vi "Duty Cycle Absolute Encoder.vi"() -> ()   [LabVIEW 2020]
doc: "This example shows how to configure and read values from an absolute encoder that has PWM duty cycle output.\n\nIt will display the raw encoder value, absolute angle, cumulative angle, and revolutions.\n\nThis example expects a USB cable connected from your development PC to the Type B USB Jack (next to the power input) on the roboRIO."
uses:
  <vilib>/Rock Robotics/SystemInterfaces/DIO/FPGA_DIOChannel.ctl
  T-Shirt Robot LV 2020/Shared Code/TypeDefs/ENUM_Tube Wheel Positions.ctl
  T-Shirt Robot LV 2020/roboRIO Code/Type Defs/Cluster_Tube Wheel Positions.ctl
  T-Shirt Robot LV 2020/roboRIO Code/Systems/Tube Wheel/Tube Wheel_ACT.lvlib
panel:
  in  "Position Array":T1[](array[typedef])=[{"Positions"=enum."Tube Red A", "Count"=47}, {"Positions"=enum."Tube Black F", "Count"=213}, {"Positions"=enum."Tube Red E", "Count"=383}, {"Positions"=enum."Tube Black D", "Count"=557}, {"Positions"=enum."Tube Red C", "Count"=724}, {"Positions"=enum."Tube Black B", "Count"=898}]
  out "Current Positions Out":T2
  out "Total Encoder Counts":i32
  out "Total Revolution":dbl
  out "Single Revolution":dbl(knob) scale=0.0..1.0 scale format="%.2g"
  out "Revolutions":i32
  out "Singel Encoder Counts":i32
  in  "Channel":T3=enum."DIO 9"
  in  "stop":bool
  # "Set this input before running."
  # "Output information."
  # "Absolute Encoder\nDuty Cycle (PWM)"
  # "This shows wiring for a generic absolute encoder with duty cycle PWM output.  Some encoders may have G labeled as Com.  Some may have +5V labeled as +VDC."
  # "Encoder\nG (brown wire)--------\n+5V (orange wire)-----\nPWM (blue wire)------"
  # "roboRIO\nDIO-0 \nDIO-0  5V\nDIO-0  S"
  # "PWM"
  # "+5V"
  # "G"
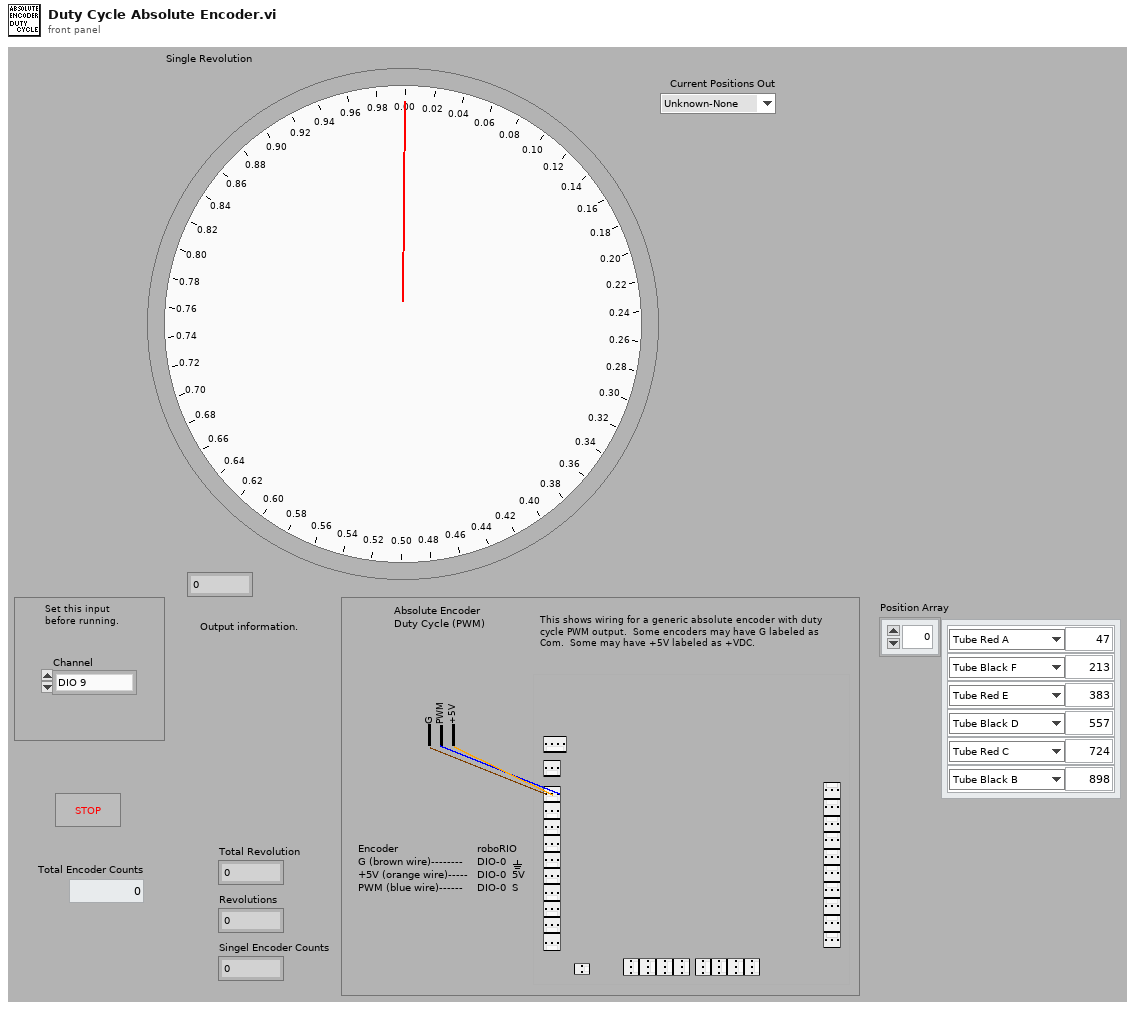
[diagram p1: front panel]
types:
  T1 = typedef "Cluster_Tube Wheel Positions.ctl" = cluster{"Positions":T2, "Count":i32}
  T2 = typedef "ENUM_Tube Wheel Positions.ctl" = enum16{"Unknown-None", "Tube Red A", "Tube Black B", "Tube Red C", "Tube Black D", "Tube Red E", "Tube Black F", "Load A-B", "Load B-C", "Load C-D", "Load D-E", "Load E-F", "Load F-A"}
  T3 = typedef "FPGA_DIOChannel.ctl" = enum8{"DIO 0", "DIO 1", "DIO 2", "DIO 3", "DIO 4", "DIO 5", "DIO 6", "DIO 7", "DIO 8", "DIO 9", "DIO MXP 0", "DIO MXP 1", "DIO MXP 2", "DIO MXP 3", "DIO MXP 4", "DIO MXP 5", "DIO MXP 6", "DIO MXP 7", "DIO MXP 8", "DIO MXP 9", "DIO MXP 10", "DIO MXP 11", "DIO MXP 12", "DIO MXP 13", "DIO MXP 14", "DIO MXP 15", "SPI Port CS1", "SPI Port CS2", "SPI Port CS3", "SPI Port MISO", "SPI Port MOSI", "Invalid"}
  T4 = typedef "Cluster_Absolute Encoder Ref.ctl" = cluster{"DutyCycleDevRef":T5, "CounterDevRef":T7}
  T5 = typedef "FPGA_DutyCycleDevRef.ctl" = cluster{"DevStatus":errorcluster, "DutyCycleIndex":T6}
  T6 = typedef "FPGA_DutyCycleIndex.ctl" = enum8{"DutyCycle 0", "DutyCycle 1", "DutyCycle 2", "DutyCycle 3", "DutyCycle 4", "DutyCycle 5", "DutyCycle 6", "DutyCycle 7", "Invalid"}
  T7 = typedef "WPI_CounterDevRef.ctl" = cluster{"DevStatus":errorcluster, "CntIndex":T8}
  T8 = typedef "FPGA_CounterCtrSystemIndex.ctl" = enum8{"Ctr 0", "Ctr 1", "Ctr 2", "Ctr 3", "Ctr 4", "Ctr 5", "Ctr 6", "Ctr 7", "Invalid"}
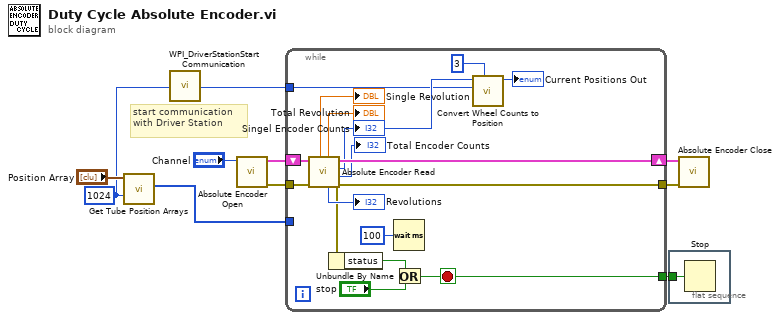
[diagram p0: block diagram]
diagram:
  w1 = 1024 ("PPR")
  # "start communication with Driver Station"
  n1 = call "Get Tube Position Arrays.vi"("PPR"=w1, "Position Array"="Position Array") -> ("Counts"=w2:i32[])  [unwired: 8 in, 1 out]
  n2 = call <vilib>:"WPI_DriverStationStart Communication.vi"() -> ()  [unwired: 3 in, 9 out]
  n3 = call "Absolute Encoder Open.vi"("Channel"="Channel") -> ("error out"=w5:errorcluster, "Cluster"=w7:T4)  [unwired: 9 in]
  n4 = while {
    shift-right: [w18] -> w6
    shift-left: w7 -> [w20]
    tunnel: [w24] -> w8
    tunnel: w5 -> [w19]
    tunnel: [w14] -> w4
    tunnel: w2 -> [_]
    tunnel: w1 -> [w10]
    stop <- w24 stop-if-true
    n5 = call "Absolute Encoder Read.vi"("Error"=w19, "Cluster"=w20) -> ("Error Out"=w14:errorcluster, "Total Encoder Counts Out"=→"Total Encoder Counts":i32, "Single Encoder Counts Out"=w13:i32, "Cluster Out"=w18:T4, "Count Out"=→"Revolutions":i32, "Total Revolution Out"=→"Total Revolution":dbl, "Single Revolution Out"=→"Single Revolution":dbl)  [unwired: 3 in]
    "Singel Encoder Counts" <- w13
    n6 = Unbundle By Name(w14) -> ("status"=w22:bool)
    n7 = Wait (ms)(milliseconds to wait=u32 100) -> ()  [unwired: 1 out]
    n8 = Or(x=w22, y="stop") -> (x .or. y?=w24:bool)
    n9 = call "Convert Wheel Counts to Position.vi"("Count Tollerance"=3, "PPR"=w10, "Wheel Count"=w13) -> ("Current Positions Out"=→"Current Positions Out":T2)  [unwired: 8 in]
  }
  n10 = flat-sequence {
    tunnel: w8 -> [w26]
    frame #0 {
      n11 = Stop(stop? (T)=w26) -> ()
    }
  }
  n12 = call "Absolute Encoder Close.vi"("Error"=w4, "Cluster"=w6) -> ()  [unwired: 10 in]
